vi "FolderCornerRectangle.vi"(8 "error out 2":errorcluster, 9 "FOLD_Y":i32, 10 "FOLD_X":i32, 11 "bounds":T2 {"height" format="%.2f"; "width" format="%.2f"; "y" format="%.2f"; "x" format="%.2f"}) -> (0 "error out":errorcluster, 2 "Array 2":T1[](array[typedef]) {"y" format="%.2f"; "x" format="%.2f"}, 3 "Array":T1[](array[typedef]) {"y" format="%.2f"; "x" format="%.2f"})   [LabVIEW 2016, in "Graphics.lvclass"]
uses:
  <resource>/Framework/Providers/Open_GDS/UML/Graphics_class/Graphics.lvclass
  <resource>/Framework/Providers/Open_GDS/UML/General/Rectangle/Rectangle Rectangle2D.ctl
  <resource>/Framework/Providers/Open_GDS/UML/General/Point/Point Point2D.ctl
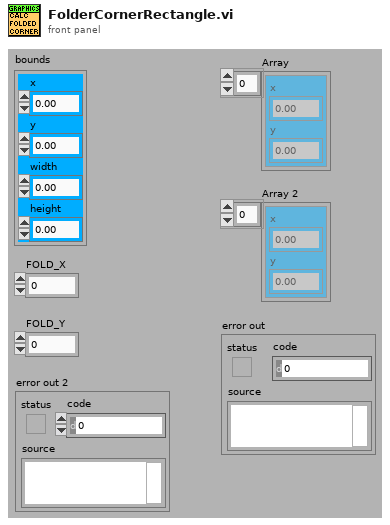
[diagram p1: front panel]
types:
  T1 = typedef "Point Point2D.ctl" = cluster{"x":dbl, "y":dbl}
  T2 = typedef "Rectangle Rectangle2D.ctl" = cluster{"x":dbl, "y":dbl, "width":dbl, "height":dbl}
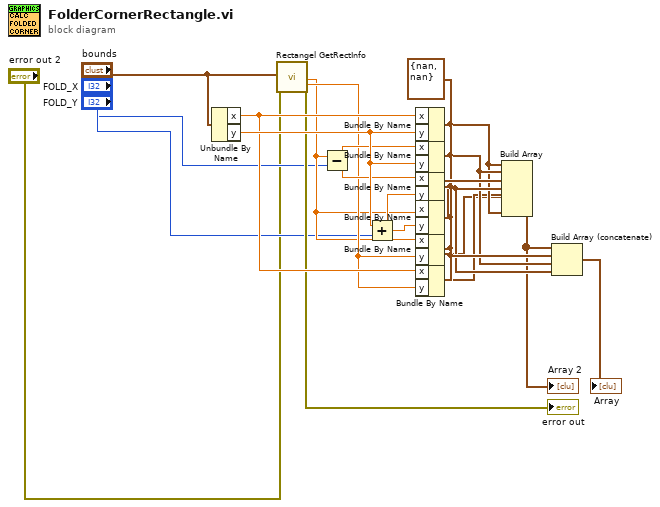
[diagram p0: block diagram]
diagram:
  w14 = T1 {"x"=nan, "y"=nan} ("point2D")
  n1 = Unbundle By Name("bounds") -> ("x"=w19:dbl, "y"=w20:dbl)
  n2 = call <resource>:"Rectangel GetRectInfo.vi"("bounds"="bounds", "error in (no error)"="error out 2") -> ("maxX"=w5:dbl, "maxY"=w10:dbl, "error out"=→"error out":errorcluster)  [unwired: 15 out]
  n3 = Subtract(x=w5, y="FOLD_X") -> (x-y=w16:dbl)
  n4 = Add(x=w20, y="FOLD_Y") -> (x+y=w17:dbl)
  n5 = Bundle By Name(cluster=w14, "x"=w19, "y"=w20) -> (w7:T1)
  n6 = Bundle By Name(cluster=w14, "x"=w16, "y"=w20) -> (w9:T1)
  n7 = Bundle By Name(cluster=w14, "x"=w16, "y"=w17) -> (w15:T1)
  n8 = Bundle By Name(cluster=w14, "x"=w5, "y"=w17) -> (w11:T1)
  n9 = Bundle By Name(cluster=w14, "x"=w5, "y"=w10) -> (w2:T1)
  n10 = Bundle By Name(cluster=w14, "x"=w19, "y"=w10) -> (w6:T1)
  n11 = Build Array(w7, w9, w15, w11, w2, w6, w7) -> (w8:T1[])
  "Array 2" <- w8
  n12 = Build Array (concatenate)(w8, w14, w9, w11) -> (→"Array":T1[])
